vi "WRIS_DataFilePath_VIG.vi"(7 "Operation":enum16{"get data", "set data"}(ring)=enum."set data", 8 "error in":errorcluster, 11 "DataFilePath_in":path) -> (0 "error out":errorcluster, 3 "DataFilePath_out":path)   [LabVIEW 2018]
doc: "VIG to store path for data file selected by operator. This is used in the UI Event loop to set, and is then Read in the Data Acq & File Loop.\n\n2008_08 Mike Ashe\nmichael.ashe@imaginatics.net"
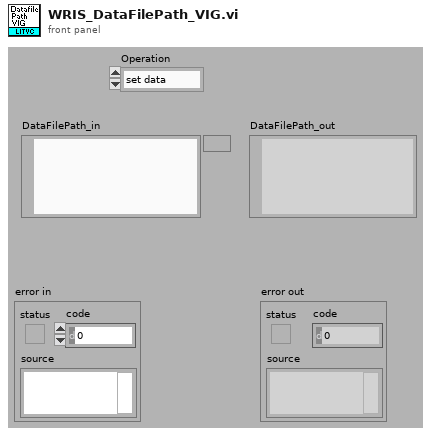
[diagram p1: front panel]
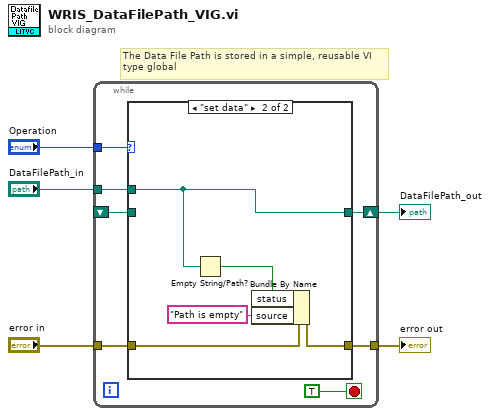
[diagram p0: block diagram]
diagram:
  # "The Data File Path is stored in a simple, reusable VI\ntype global"
  n1 = while {
    tunnel: "Operation" -> [w12]
    shift-right: [w10] -> w3
    shift-left: _ -> [w8]
    tunnel: "DataFilePath_in" -> [w9]
    tunnel: "error in" -> [w7]
    tunnel: [w6] -> w1
    stop <- TRUE stop-if-true
    n2 = case shown="\"set data\"" w12 {
      tunnel: [w14 w16] -> w10
      tunnel: w9 -> [_ w16]
      tunnel: w8 -> [w14 _]
      tunnel: w7 -> [w13 w19]
      tunnel: [w13 w18] -> w6
      frame "get data", Default {
      }
      frame "set data" {
        n3 = Empty String/Path?(string/path=w16) -> (empty?=w15:bool)
        n4 = Bundle By Name(cluster=w19, "status"=w15, "source"="Path is empty") -> (w18:errorcluster)
      }
    }
  }
  "error out" <- w1
  "DataFilePath_out" <- w3
